vi "threshold-double.vi"(10 "Search":dbl=nan format="%#_13g", 11 "Data (dbl) []":dbl[](array[numeric])) -> (3 "Index":dbl format="%.2f")   [LabVIEW 2015, in "binary_search.lvlib"]
uses:
  binary_search.lvlib
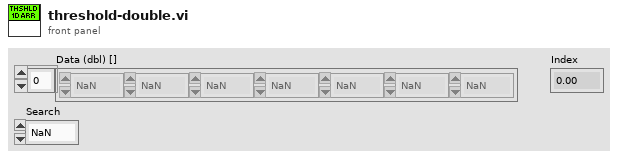
[diagram p1: front panel]
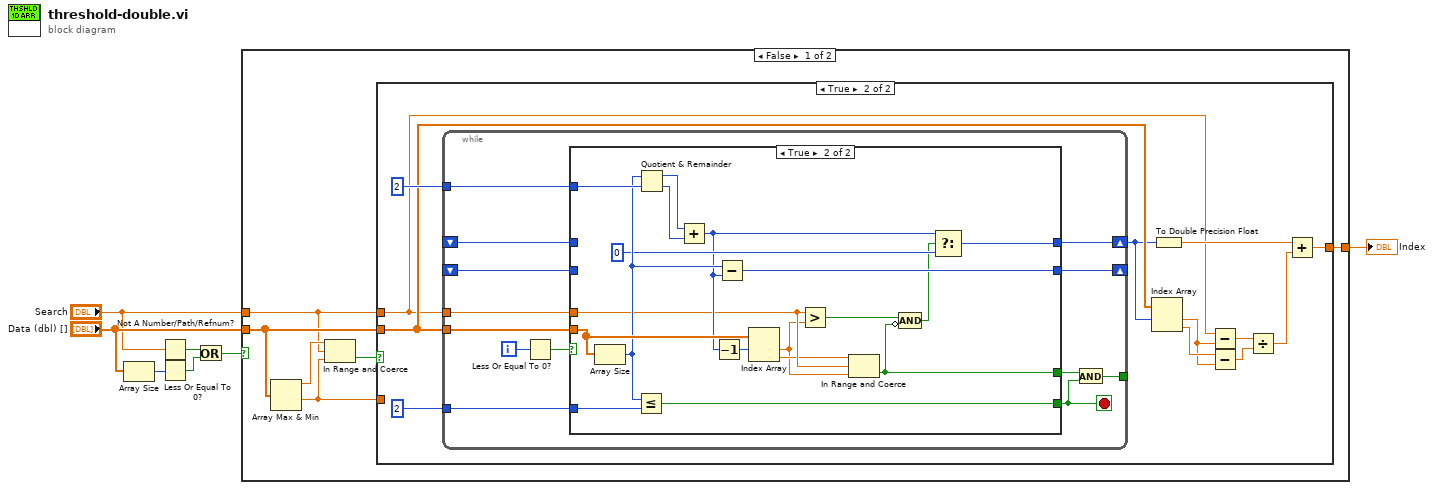
[diagram p0: block diagram]
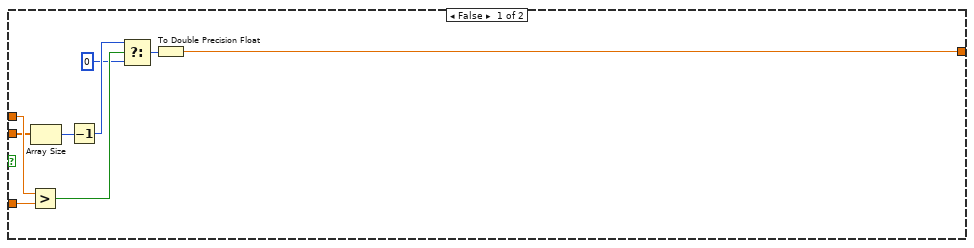
[diagram p2: hidden frame]
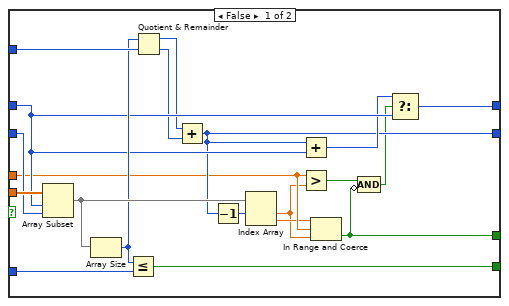
[diagram p3: hidden frame]
diagram:
  n1 = Array Size(array="Data (dbl) []") -> (size(s)=w3:i32)
  n2 = Not A Number/Path/Refnum?(number/path/refnum="Search") -> (NaN/Path/Refnum?=w7:bool)
  n3 = Less Or Equal To 0?(x=w3) -> (x <= 0?=w6:bool)
  n4 = Or(x=w7, y=w6) -> (x .or. y?=w2:bool)
  n5 = case shown="False" w2 {
    tunnel: "Data (dbl) []" -> [w12 _]
    tunnel: "Search" -> [w10 _]
    tunnel: [w13 _] -> w1
    frame False {
      n6 = Array Max & Min(array=w12) -> (max value=w11:dbl, min value=w8:dbl)  [unwired: 2 out]
      n7 = In Range and Coerce(upper limit=w11, x=w10, lower limit=w8) -> (In Range?=w9:bool)  [unwired: 1 out]
      n8 = case shown="True" w9 {
        tunnel: [w14 w29] -> w13
        tunnel: w12 -> [w21 w25]
        tunnel: w10 -> [w22 w24]
        tunnel: w8 -> [w19 _]
        frame False {
          n9 = Greater?(x=w22, y=w19) -> (0:w18:bool)
          n10 = Array Size(array=w21) -> (size(s)=w20:i32)
          n11 = Decrement(x=w20) -> (x-1=w17:i32)
          n12 = Select(t=w17, s=w18, f=0) -> (s? t:f=w15:i32)
          n13 = To Double Precision Float(number=w15) -> (double precision float=w14:dbl)
        }
        frame True {
          n14 = while {
            tunnel: w25 -> [w45]
            tunnel: w24 -> [w47]
            shift-right: [w44] -> w23
            shift-left: _ -> [w46]
            shift-right: [w43] -> _
            shift-left: _ -> [w42]
            tunnel: 2 ("y") -> [w39]
            tunnel: 2 ("y") -> [w38]
            tunnel: [w35] -> _
            i -> [w41]
            stop <- w36 stop-if-true
            n15 = Less Or Equal To 0?(x=w41) -> (x <= 0?=w40:bool)
            n16 = case shown="True" w40 {
              tunnel: w47 -> [w53 w73]
              tunnel: w46 -> [w59 _]
              tunnel: w45 -> [w67 w85]
              tunnel: [w63 w83] -> w44
              tunnel: [w56 w84] -> w43
              tunnel: w42 -> [w66 _]
              tunnel: [w55 w74] -> w36
              tunnel: w39 -> [w64 w82]
              tunnel: w38 -> [w62 w81]
              tunnel: [w50 w70] -> w37
              frame False {
                n17 = Array Subset(array=w67, index=w59, length=w66) -> (w65:dbl[])
                n18 = Array Size(array=w65) -> (size(s)=w61:i32)
                n19 = Less Or Equal?(x=w61, y=w64) -> (x <= y?=w55:bool)
                n20 = Quotient & Remainder(x=w61, y=w62) -> (x-y*floor(x/y)=w57:i32, floor(x/y)=w54:i32)
                n21 = Add(x=w57, y=w54) -> (x+y=w56:i32)
                n22 = Decrement(x=w56) -> (x-1=w60:i32)
                n23 = Index Array(array=w65, index #1=w60) -> (element #1=w51:dbl, element #2=w52:dbl)  [unwired: 1 in]
                n24 = Add(x=w56, y=w59) -> (x+y=w58:i32)
                n25 = Greater?(x=w53, y=w51) -> (0:w49:bool)
                n26 = In Range and Coerce(upper limit=w52, x=w53, lower limit=w51) -> (In Range?=w50:bool)  [unwired: 1 out]
                n27 = Compound Arithmetic op=AND(w49, invert w50) -> (w48:bool)
                n28 = Select(t=w58, s=w48, f=w59) -> (s? t:f=w63:i32)
              }
              frame True {
                n29 = Array Size(array=w85) -> (size(s)=w80:i32)
                n30 = Less Or Equal?(x=w80, y=w82) -> (x <= y?=w74:bool)
                n31 = Quotient & Remainder(x=w80, y=w81) -> (x-y*floor(x/y)=w75:i32, floor(x/y)=w77:i32)
                n32 = Add(x=w75, y=w77) -> (x+y=w76:i32)
                n33 = Decrement(x=w76) -> (x-1=w78:i32)
                n34 = Subtract(x=w80, y=w76) -> (x-y=w84:i32)
                n35 = Index Array(array=w85, index #1=w78) -> (element #1=w71:dbl, element #2=w72:dbl)  [unwired: 1 in]
                n36 = Greater?(x=w73, y=w71) -> (0:w69:bool)
                n37 = In Range and Coerce(upper limit=w72, x=w73, lower limit=w71) -> (In Range?=w70:bool)  [unwired: 1 out]
                n38 = Compound Arithmetic op=AND(w69, invert w70) -> (w68:bool)
                n39 = Select(t=w76, s=w68, f=0) -> (s? t:f=w83:i32)
              }
            }
            n40 = And(x=w37, y=w36) -> (x .and. y?=w35:bool)
          }
          n41 = Index Array(array=w25, index #1=w23) -> (element #1=w33:dbl, element #2=w34:dbl)  [unwired: 1 in]
          n42 = To Double Precision Float(number=w23) -> (double precision float=w28:dbl)
          n43 = Subtract(x=w24, y=w33) -> (x-y=w32:dbl)
          n44 = Subtract(x=w34, y=w33) -> (x-y=w31:dbl)
          n45 = Divide(x=w32, y=w31) -> (x/y=w30:dbl)
          n46 = Add(x=w28, y=w30) -> (x+y=w29:dbl)
        }
      }
    }
    frame True {
    }
  }
  "Index" <- w1
